vi "Queue remove.vi"(9 "output cluster":T1) -> (1 "output cluster 2":T1, 3 "Message Cluster":T2)   [LabVIEW 2015]
uses:
  QMH Fundamentals - Message Cluster.ctl
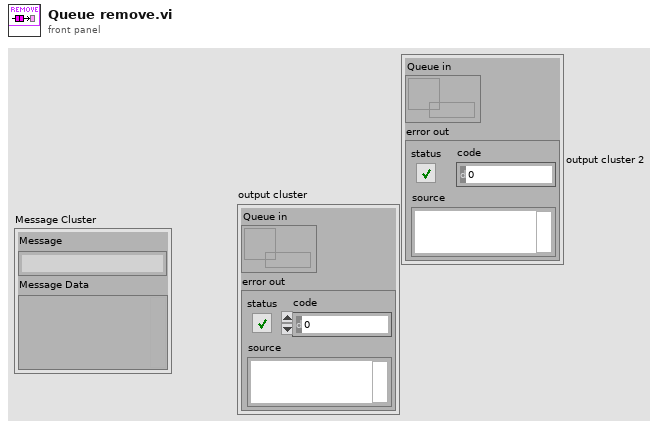
[diagram p1: front panel]
types:
  T1 = cluster{"Queue in":refnum<queue>, "error out":errorcluster}
  T2 = typedef "QMH Fundamentals - Message Cluster.ctl" = cluster{"Message":string, "Message Data":variant}
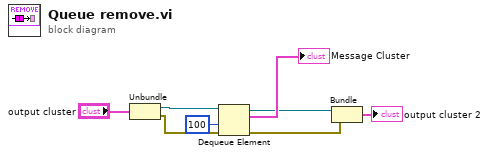
[diagram p0: block diagram]
diagram:
  n1 = Unbundle("output cluster") -> ("Queue in"=w4:refnum<queue>, "error out"=w3:errorcluster)
  n2 = Dequeue Element(queue=w4, timeout in ms (-1)=100, error in (no error)=w3) -> (queue out=w7:refnum<queue>, element=→"Message Cluster":T2, error out=w6:errorcluster)  [unwired: 1 out]
  n3 = Bundle("Queue in"=w7, "error out"=w6) -> (→"output cluster 2":T1)  [unwired: 1 in]
